vi "Launch Logger.vi"(8 "error in (no error)":errorcluster, 11 "DataProcessor in":refnum<class "DataProcessor.lvclass">) -> (0 "error out":errorcluster, 3 "DataProcessor out":refnum<class "DataProcessor.lvclass">)   [LabVIEW 2020, in "Volatus.lvlib" / "DataProcessor.lvclass"]
uses:
  DataProcessor.lvclass
  C:/dev/lv20CE/relink/lv-volatus/Volatus/DataHandlerTask/DataHandlerTask.lvclass
  C:/dev/lv20CE/relink/lv-volatus/Volatus/Task/Task.lvclass
  DataHandlerAPI/DataHandlerAPI.lvclass
  C:/dev/lv20CE/relink/lv-volatus/Volatus/API/API.lvclass
  DataLogger/DataLogger.lvclass
  DataProcessor.lvclass/DataProcessor.ctl
  DataHandlerTask/DataHandlerTask.lvclass/DataHandlerTask.ctl
  VolatusConfig/VolatusConfigElement/VolatusConfigElement.lvclass/VolatusConfigElement.ctl
  VolatusConfig/VolatusConfigElement/Element.vi
  VolatusConfig/Task/Task.lvclass
  C:/dev/lv20CE/relink/lv-volatus/VolatusConfig/VolatusConfigElement/VolatusConfigElement.lvclass
  Task/Task.lvclass
  VolatusConfig/VolatusConfigElement/VolatusConfigElement.lvclass
  DataHandlerTask/DataHandlerTask.lvclass
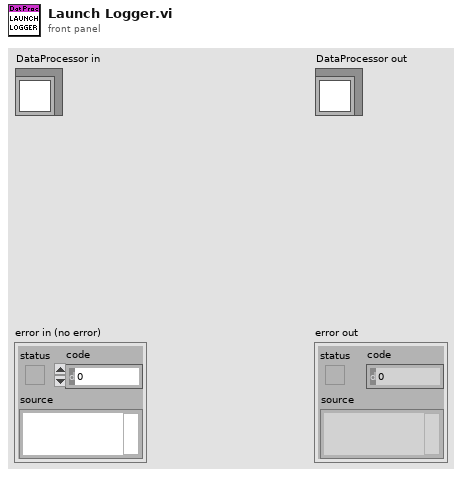
[diagram p1: front panel]
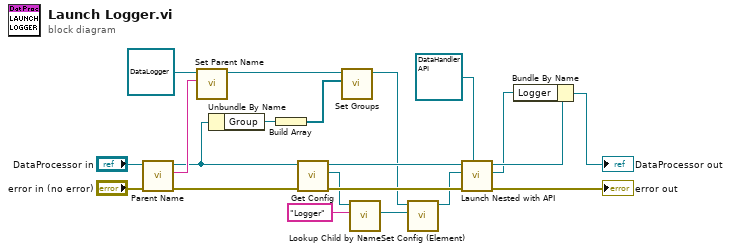
[diagram p0: block diagram]
diagram:
  n1 = call "Parent Name.vi"("error in (no error)"="error in (no error)", "DataHandlerTask in"="DataProcessor in") -> ("error out"=w8:errorcluster, "Parent Name"=w6:string, "DataHandlerTask out"=w3:refnum<class "DataProcessor.lvclass">)  [unwired: 7 in]
  n2 = call "Set Parent Name.vi"("Parent Name"=w6, "DataHandlerTask in"=refnum<class "DataLogger.lvclass"> refnum ("Volatus:DataLogger.lvclass")) -> ("DataHandlerTask out"=w9:refnum<class "DataLogger.lvclass">)  [unwired: 8 in, 1 out]
  n3 = Unbundle By Name(w3) -> ("Group"=w2:refnum<class "Group.lvclass">)
  n4 = Build Array(w2) -> (w1:refnum<class "Group.lvclass">[])
  n5 = call "Get Config.vi"("error in (no error)"=w8, "Task in"=w3) -> ("error out"=w20:errorcluster, "Config"=w19:refnum<class "Task.lvclass">, "Task out"=w15:refnum<class "DataProcessor.lvclass">)  [unwired: 7 in]
  n6 = call "Set Groups.vi"("Groups"=w1, "DataLogger in"=w9) -> ("DataLogger out"=w4:refnum<class "DataLogger.lvclass">)  [unwired: 8 in, 1 out]
  n7 = call "Lookup Child by Name.vi"("Child Name"="Logger", "VolatusConfigElement in"=w19) -> ("Child"=w17:refnum<class "Config Element.lvclass">)  [unwired: 6 in, 3 out]
  n8 = call "Set Config (Element).vi"("Config Element"=w17, "Task in"=w4) -> ("Task out"=w13:refnum<class "DataLogger.lvclass">)  [unwired: 8 in, 1 out]
  n9 = call "Launch Nested with API.vi"("API Type"=refnum<class "DataHandlerAPI.lvclass"> refnum ("Volatus:DataHandlerAPI"), "error in (no error)"=w20, "Nested Task"=w13, "Task in"=w15) -> ("error out"=→"error out":errorcluster, "API"=w5:refnum<class "DataHandlerAPI.lvclass">, "Task out"=w14:refnum<class "DataProcessor.lvclass">)  [unwired: 5 in]
  n10 = Bundle By Name(cluster=w14, "Logger"=w5) -> (→"DataProcessor out":refnum<class "DataProcessor.lvclass">)
